vi "Read Websocket Client Handler.vi"(11 "Websocket Server in":refnum<class "Websocket Server.lvclass">) -> (2 "Stream Mediator.lvlib:Websocket Client Handler.lvclass":refnum<class "Websocket Client Handler.lvclass">, 3 "Websocket Server out":refnum<class "Websocket Server.lvclass">)   [LabVIEW 2016, in "Stream Mediator.lvlib" / "Websocket Server.lvclass"]
uses:
  <userlib>/Composed Systems/Stream/Mediator/Classes/Websocket Server Actor/Websocket Server/Websocket Server.lvclass
  <userlib>/Composed Systems/Stream/Mediator/Classes/Websocket Client Handler Actor/Websocket Client Handler/Websocket Client Handler.lvclass
  <userlib>/Composed Systems/Stream/Mediator/Classes/Websocket Server Actor/Websocket Server/Websocket Server.lvclass/Websocket Server.ctl
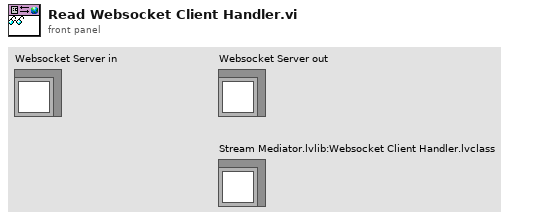
[diagram p1: front panel]
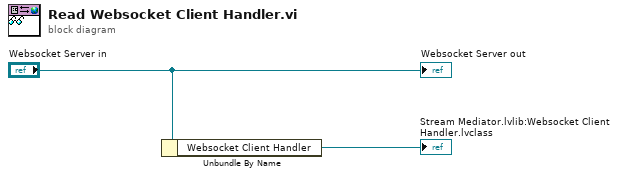
[diagram p0: block diagram]
diagram:
  n1 = Unbundle By Name("Websocket Server in") -> ("Websocket Client Handler"=→"Stream Mediator.lvlib:Websocket Client Handler.lvclass":refnum<class "Websocket Client Handler.lvclass">)
  "Websocket Server out" <- "Websocket Server in"
